vi "New Problem Template.vi"() -> ()   [LabVIEW 2021, in "Project Euler.lvlib"]
uses:
  Project Euler.lvlib
  Utilities/Named Timers/Named Timers.lvlib
panel:
  out "Answer":string
  out "Total execution time (ms)":u32
  # "Development\nControls or indicators that are useful for development or testing, but which are not outputs of the VI."
  # "Input\nInputs to the VI"
  # "Output\nOutputs of the VI"
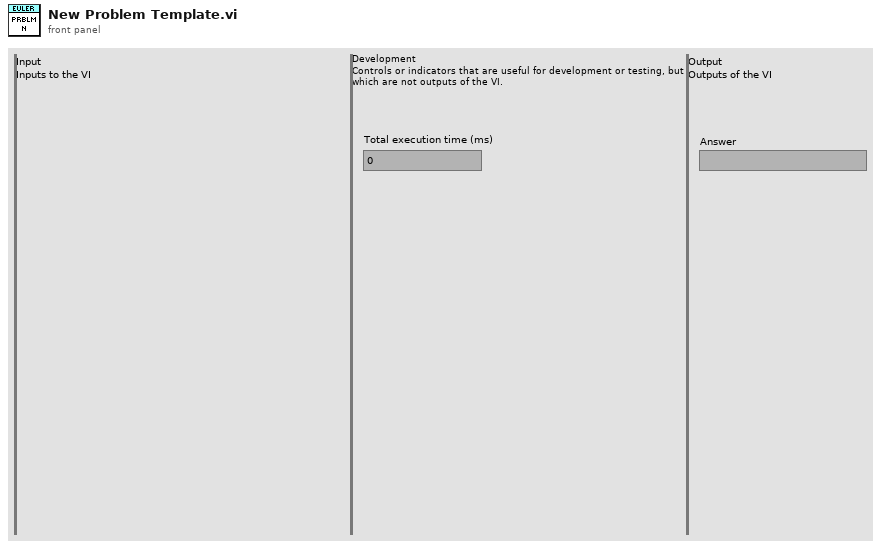
[diagram p1: front panel]
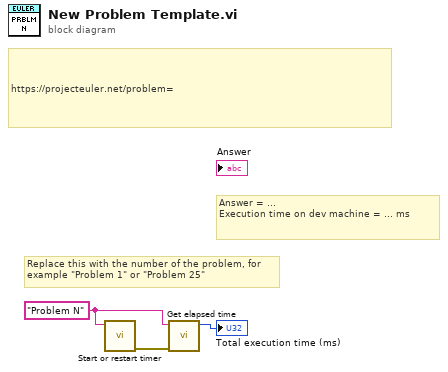
[diagram p0: block diagram]
diagram:
  w1 = "Problem N" ("Timer name")
  # "Replace this with the number of the problem, for example \"Problem 1\" or \"Problem 25\""
  # "Answer = ... \nExecution time on dev machine = ... ms"
  # "https://projecteuler.net/problem="
  n1 = call "Start or restart timer.vi"("Timer name"=w1) -> ("error out"=w2:errorcluster)  [unwired: 10 in]
  n2 = call "Get elapsed time.vi"("error in (no error)"=w2, "Timer name"=w1) -> ("Elapsed time (ms)"=→"Total execution time (ms)":u32)  [unwired: 6 in, 3 out]
